vi "SMO.InstrumentDriver.MeasureValue.vi"(8 "error in (no error)":errorcluster, 11 "SMO.Instrument":refnum<class "SMO.InstrumentDriver.lvclass">) -> (0 "error out":errorcluster, 2 "value":T1, 3 "SMO.Instrument out":refnum<class "SMO.InstrumentDriver.lvclass">)   [LabVIEW 2013, in "SMO.InstrumentDriver.lvclass"]
doc: "---------------------------------------------------------------\nJKI State Machine Objects™\nhttp://jki.net/state-machine-objects/\nCopyright (C) 2005-2015, JKI <info@jki.net>\nALL RIGHTS RESERVEDJKI State Machine Objects (SMO) 1.0.0.5\nJKI - JKI\nCopyright (c) 2016, JKI"
uses:
  SMO.InstrumentDriver.lvclass
  Typedefs/Data.ctl
panel:
  # "For instructions on how to use the JKI State Machine Objects, examples and video tutorials, visit:\nhttp://jki.net/state-machine-objects/\n\nJKI State Machine Objects™\nhttp://jki.net/state-machine-objects/\nCopyright (C) 2005-2015, JKI <info@jki.net>\nALL RIGHTS RESERVED"
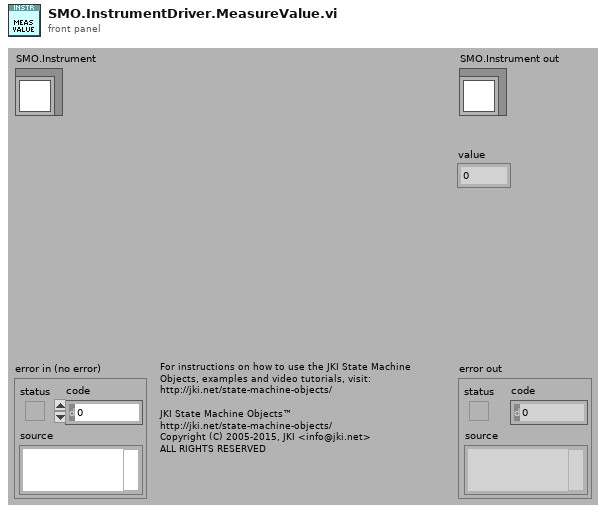
[diagram p1: front panel]
types:
  T1 = typedef "SMO.InstrumentDriver.lvclass/Data.ctl" = dbl
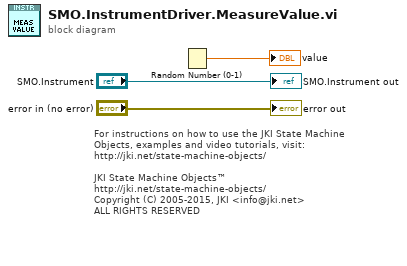
[diagram p0: block diagram]
diagram:
  # "For instructions on how to use the JKI State Machine Objects, examples and video tutorials, visit:\nhttp://jki.net/state-machine-objects/\n\nJKI State Machine Objects™\nhttp://jki.net/state-machine-objects/\nCopyright (C) 2005-2015, JKI <info@jki.net>\nALL RIGHTS RESERVED"
  n1 = Random Number (0-1)() -> (number: 0 to 1=→"value":dbl)
  "error out" <- "error in (no error)"
  "SMO.Instrument out" <- "SMO.Instrument"
